vi "multi_sensor.vi"() -> ()   [LabVIEW 2012]
uses:
  <vilib>/Instr/_visa.llb/VISA Configure Serial Port (Instr).vi
panel:
  out "date2":string
  out "Time2":string
  in  "Heart rate":path
  out "power":dbl(slide) scale=0.0..200.0
  out "1":u32
  out "read buffer 2":string
  out "2":u32
  in  "Blank Button":bool
  out "read buffer":string
  out "Time":string
  out "Date":string
  out "Temprature Value":dbl
  out "Heart Rate":dbl
  out "Temprature":dbl(slide) scale=0.0..100.0
  out "?":dbl(knob) scale=0.0..140.0
  in  "Temp":path
  in  "VISA resource name":refnum<visa-resource-name>
  in  "Stop Button":bool
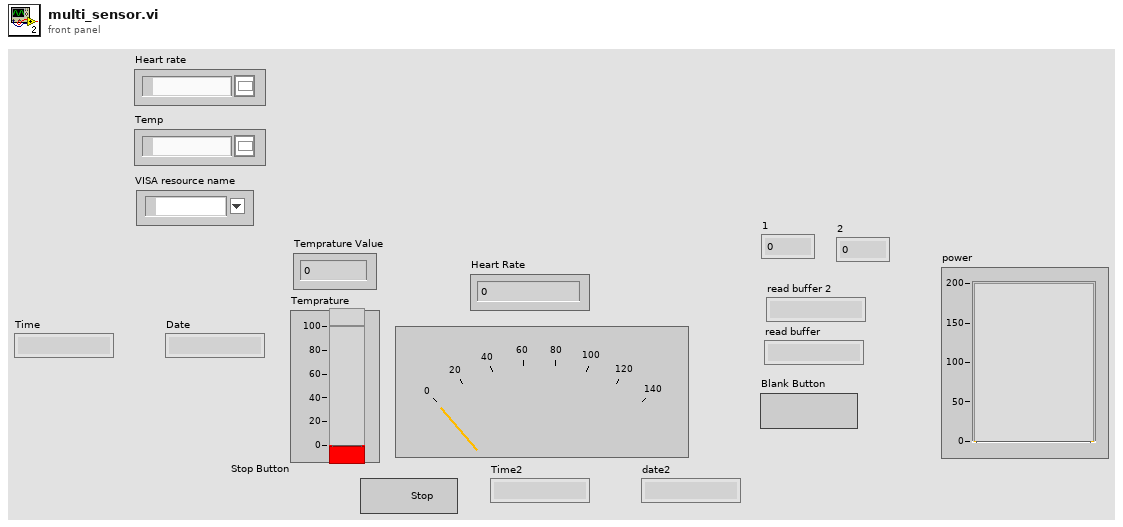
[diagram p1: front panel]
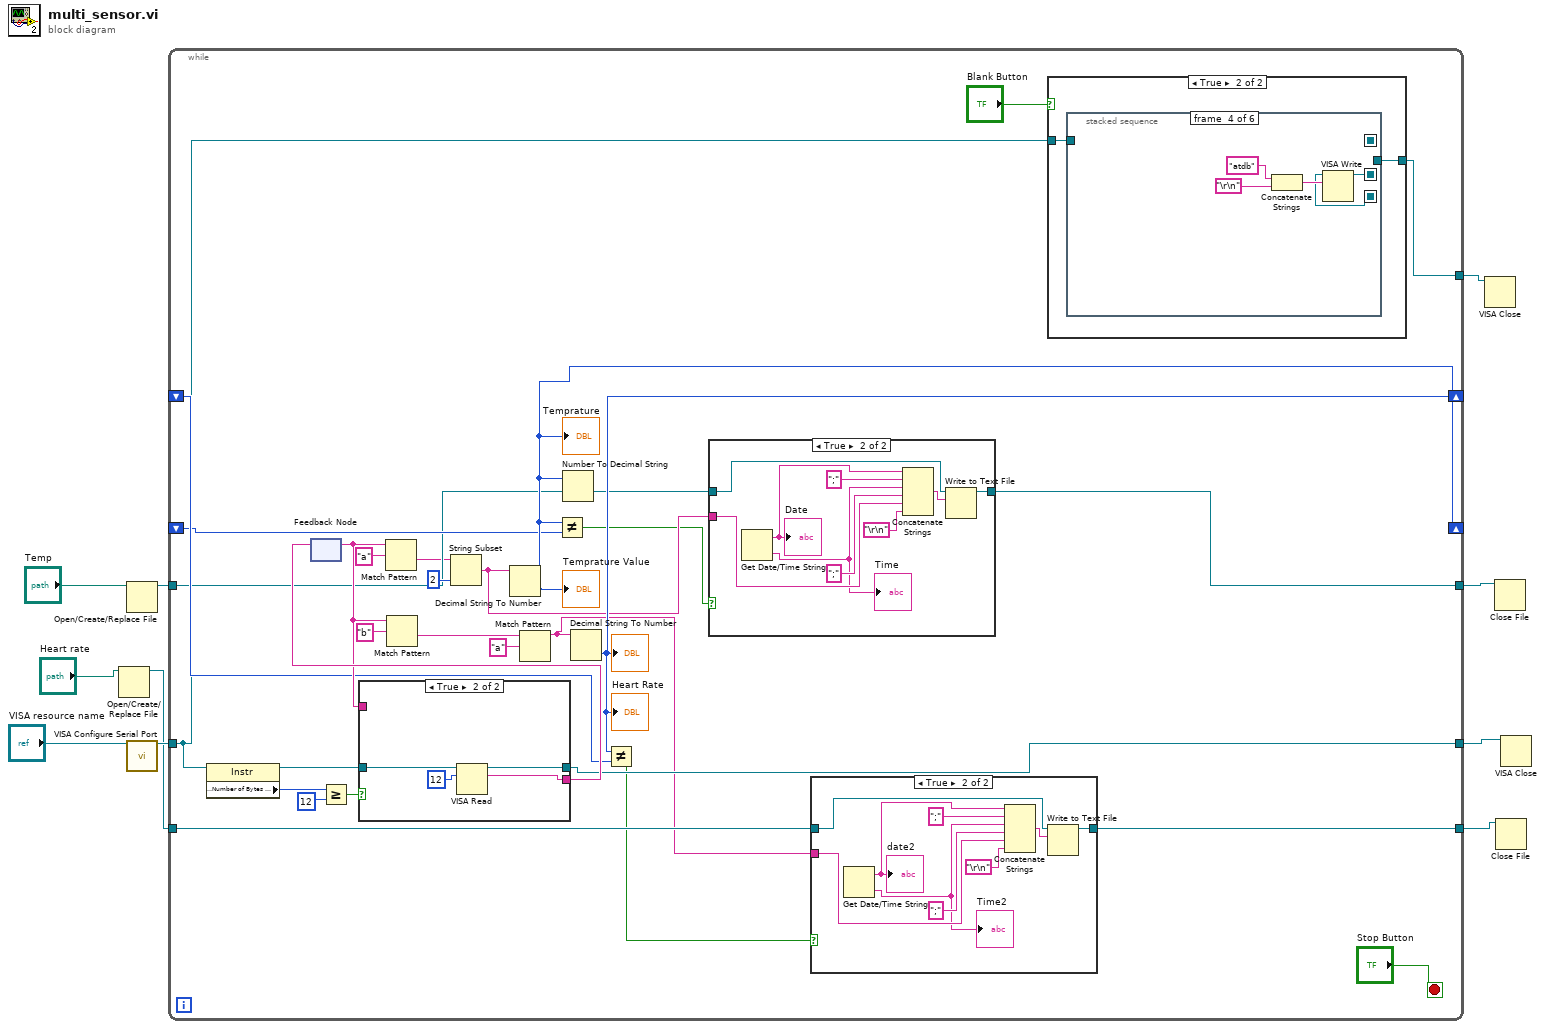
[diagram p0: block diagram]
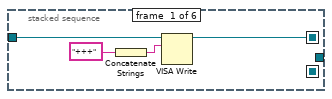
[diagram p4: hidden frame]
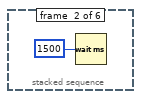
[diagram p5: hidden frame]
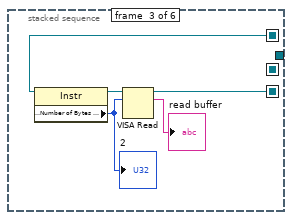
[diagram p6: hidden frame]
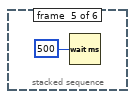
[diagram p7: hidden frame]
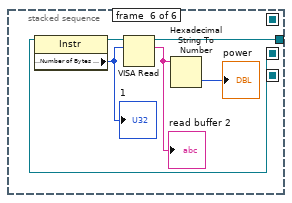
[diagram p8: hidden frame]
diagram:
  n1 = Open/Create/Replace File(file path (use dialog)="Heart rate") -> (refnum out=w2:refnum<file>)  [unwired: 5 in, 2 out]
  n2 = Open/Create/Replace File(file path (use dialog)="Temp") -> (refnum out=w7:refnum<file>)  [unwired: 5 in, 2 out]
  n3 = call-poly "VISA Configure Serial Port"("VISA resource name"="VISA resource name") -> ("VISA resource name out"=w10:refnum<visa-resource-name>)  [unwired: 13 in, 1 out]
  n4 = while {
    tunnel: w10 -> [w18]
    tunnel: [w29] -> w9
    tunnel: w7 -> [w23]
    tunnel: [w24] -> w6
    shift-right: [w28] -> _
    shift-left: _ -> [w26]
    shift-right: [w27] -> _
    shift-left: _ -> [w25]
    tunnel: [w17] -> w4
    tunnel: w2 -> [w15]
    tunnel: [w11] -> w1
    stop <- "Stop Button" stop-if-true
    n5 = property class="Instr"(reference=w18) -> (reference out=w35:refnum<visa-resource-name>, "Serial Settings:Number of Bytes at Serial Port"=w32:u32)  [unwired: 1 in, 1 out]
    n6 = feedback #1() -> (w33:string)  [unwired: 1 in]
    n7 = Greater Or Equal?(x=w32, y=u32 12) -> (x >= y?=w30:bool)
    n8 = case shown="True" w30 {
      tunnel: [w85 w90] -> w34
      tunnel: w35 -> [w86 w89]
      tunnel: [w86 w88] -> w29
      tunnel: w33 -> [w85 _]
      frame False {
      }
      frame True {
        n9 = VISA Read(VISA resource name=w89, byte count=u32 12) -> (VISA resource name out=w88:refnum<visa-resource-name>, read buffer=w90:string)  [unwired: 1 in, 2 out]
      }
    }
    n10 = feedback-in #1(w34) -> ()
    n11 = Match Pattern(string=w33, regular expression="a") -> (after substring=w22:string)  [unwired: 1 in, 3 out]
    n12 = Match Pattern(string=w33, regular expression="b") -> (after substring=w20:string)  [unwired: 1 in, 3 out]
    n13 = String Subset(string=w22, length (rest)=2 ("length (rest)")) -> (substring=w21:string)  [unwired: 1 in]
    n14 = Decimal String To Number(string=w21) -> (number=w27:i32)  [unwired: 2 in, 1 out]
    "Temprature" <- w27
    "Temprature Value" <- w27
    n15 = Match Pattern(string=w20, regular expression="a") -> (before substring=w14:string)  [unwired: 1 in, 3 out]
    n16 = Not Equal?(x=w27, y=w25) -> (x != y?=w13:bool)
    n17 = Number To Decimal String(number=w27) -> ()  [unwired: 1 in, 1 out]
    n18 = Decimal String To Number(string=w14) -> (number=w28:i32)  [unwired: 2 in, 1 out]
    "?" <- w28
    "Heart Rate" <- w28
    n19 = Not Equal?(x=w28, y=w26) -> (x != y?=w12:bool)
    n20 = case shown="True" w13 {
      tunnel: [w75 w84] -> w24
      tunnel: w23 -> [w75 w83]
      tunnel: w21 -> [_ w79]
      frame False {
      }
      frame True {
        n21 = Get Date/Time String() -> (date string=w82:string, time string=w77:string)  [unwired: 3 in]
        "Date" <- w82
        "Time" <- w77
        n22 = Concatenate Strings(w82, ";" ("string"), w77, ";" ("string"), w79, "\r\n") -> (w78:string)
        n23 = Write to Text File(file (use dialog)=w83, text=w78) -> (refnum out=w84:refnum<file>)  [unwired: 2 in, 2 out]
      }
    }
    n24 = case shown="True" w12 {
      tunnel: [w40 w49] -> w11
      tunnel: w15 -> [w40 w48]
      tunnel: w14 -> [_ w44]
      frame False {
      }
      frame True {
        n25 = Get Date/Time String() -> (date string=w47:string, time string=w42:string)  [unwired: 3 in]
        "date2" <- w47
        "Time2" <- w42
        n26 = Concatenate Strings(w47, ";" ("string"), w42, ";" ("string"), w44, "\r\n") -> (w43:string)
        n27 = Write to Text File(file (use dialog)=w48, text=w43) -> (refnum out=w49:refnum<file>)  [unwired: 2 in, 2 out]
      }
    }
    n28 = case shown="True" "Blank Button" {
      tunnel: w18 -> [w50 w52]
      tunnel: [w50 w51] -> w17
      frame False {
      }
      frame True {
        n29 = stacked-sequence {
          seq-local: [w53 _ _ _ _ _] -> [_ _ w60 _ _ _]
          seq-local: [_ _ w58 _ _ _] -> [_ _ _ w65 _ _]
          seq-local: [_ _ _ w63 _ _] -> [_ _ _ _ _ w72]
          tunnel: w52 -> [w56 _ _ _ _ _]
          tunnel: [_ _ _ _ _ w71] -> w51
          frame #0 {
            n30 = Concatenate Strings("+++" ("string")) -> (w54:string)
            n31 = VISA Write(VISA resource name=w56, write buffer=w54) -> (VISA resource name out=w53:refnum<visa-resource-name>)  [unwired: 1 in, 2 out]
          }
          frame #1 {
            n32 = Wait (ms)(milliseconds to wait=u32 1500) -> ()  [unwired: 1 out]
          }
          frame #2 {
            n33 = property class="Instr"(reference=w60) -> (reference out=w59:refnum<visa-resource-name>, "Serial Settings:Number of Bytes at Serial Port"=w62:u32)  [unwired: 1 in, 1 out]
            "2" <- w62
            n34 = VISA Read(VISA resource name=w59, byte count=w62) -> (VISA resource name out=w58:refnum<visa-resource-name>, read buffer=→"read buffer":string)  [unwired: 1 in, 2 out]
          }
          frame #3 {
            n35 = Concatenate Strings("atdb" ("string"), "\r\n") -> (w66:string)
            n36 = VISA Write(VISA resource name=w65, write buffer=w66) -> (VISA resource name out=w63:refnum<visa-resource-name>)  [unwired: 1 in, 2 out]
          }
          frame #4 {
            n37 = Wait (ms)(milliseconds to wait=u32 500) -> ()  [unwired: 1 out]
          }
          frame #5 {
            n38 = property class="Instr"(reference=w72) -> (reference out=w73:refnum<visa-resource-name>, "Serial Settings:Number of Bytes at Serial Port"=w74:u32)  [unwired: 1 in, 1 out]
            "1" <- w74
            n39 = VISA Read(VISA resource name=w73, byte count=w74) -> (VISA resource name out=w71:refnum<visa-resource-name>, read buffer=w70:string)  [unwired: 1 in, 2 out]
            "read buffer 2" <- w70
            n40 = Hexadecimal String To Number(string=w70) -> (number=→"power":u32)  [unwired: 2 in, 1 out]
          }
        }
      }
    }
  }
  n41 = VISA Close(VISA resource name=w4) -> ()  [unwired: 1 in, 1 out]
  n42 = Close File(refnum=w6) -> ()  [unwired: 1 in, 2 out]
  n43 = Close File(refnum=w1) -> ()  [unwired: 1 in, 2 out]
  n44 = VISA Close(VISA resource name=w9) -> ()  [unwired: 1 in, 1 out]
